vi "Soft_Robot_Model_Conf.vi"() -> ()   [LabVIEW 2015]
uses:
  <vilib>/addons/Control Design/_Stochastic Systems/Stochastic Systems.llb/Stochastic Systems SubVIs/cd_Stochastic State-Space Model.ctl
  <vilib>/addons/Control Design/_Model Construction/Model Typedefs.llb/CD State Space Model (MIMO).ctl
  <vilib>/addons/Control Design/_Model Construction/Model Typedefs.llb/CD General Elements.ctl
  <vilib>/addons/Control Design/_Stochastic Systems/Stochastic Systems.llb/CD CtoD Stochastic Model.ctl
  <vilib>/Platform/TimedLoop/XDataNode/timing_clust.ctl
  <vilib>/Platform/TimedLoop/XDataNode/nitl_modes.ctl
  <vilib>/Platform/TimedLoop/XDataNode/wakeup.ctl
  <vilib>/addons/Control Design/_Stochastic Systems/Stochastic Systems.llb/CD Construct Stochastic Model (Numeric).vi
  <vilib>/FPGAPlugInAG/myRIO-1900/niLvFpga_Open_myRIO-1900.vi
  <vilib>/rvi/interface/common/dynamic/niFpgaDynamicAddResources.vi
  <vilib>/Utility/error.llb/Error Cluster From Error Code.vi
  <vilib>/rvi/errors/niLvFpgaAdjustHostInterfaceError.vi
  <vilib>/FPGAPlugInAG/Dynamic/niLvFpga_Close_Dynamic.vi
  <vilib>/Analysis/7linalg.llb/Create Special Real Matrix.vi
  <vilib>/addons/Control Design/_Stochastic Systems/Stochastic Systems.llb/CD Construct Noise Model (Numeric).vi
  <vilib>/addons/Control Design/_State Feedback Control/State Feedback Control.llb/State Feedback Control SubVis/cd_Linear Quadratic Regulator.vi
  <vilib>/Simulation/Estimation/Implementation/NILVSim Discrete Kalman Filter.llb/SIM Disc KF Pred and Corr with Pred Gain with Checking Direct LV.vi
  <vilib>/Simulation/DiscreteLinear/Implementation/NILVSim Discrete Stochastic State Space.llb/NILVSim Discrete Stochastic State Space Internal Direct LV.vi
  <vilib>/addons/Control Design/_Implementation/CD State Feedback Controller (Multiple Outputs).vi
  <vilib>/Platform/TimedLoop/XDataNode/XDataNode.xnode
  <vilib>/rvi/interface/nirviOpenFPGA/nirviOpenFPGA.xnode
  FPGA Bitfiles/ACC20115_FPGATarget_CurrentControlle_Dt5vFgOzYtY.lvbitx
  Current Controller.vi
  <vilib>/rvi/interface/nirviReadWriteControl/nirviReadWriteControl.xnode
  <vilib>/rvi/interface/nirviCloseFPGA/nirviCloseFPGA.xnode
  <vilib>/Simulation/Implementation/XNodeFramework/SimXNode/SimX.xnode
  <vilib>/addons/Control Design/_State Feedback Control/NI_CD_State Feedback Control.lvlib
  <vilib>/Analysis/NI_AALPro.lvlib
  <vilib>/Platform/TimedLoop/XDataNode/XDNodeRunTimeDep.lvlib
  <vilib>/rvi/interface/Simulation/niFpgaSimulationCallBeginRW.vi
  <vilib>/addons/Control Design/_Stochastic Systems/NI_CD_Stochastic Systems.lvlib
  <vilib>/addons/Control Design/_State-Space Analysis/NI_CD_State-Space Analysis.lvlib
  NiFpgaLv.dll
  <vilib>/addons/Control Design/_Implementation/NI_CD_Implementation.lvlib
  <vilib>/addons/Control Design/_Model Construction/NI_LinSys_Model Typedefs.lvlib
panel:
  in  "SP":dbl(slide) scale=580.0..720.0
  in  "Tab Control":enum32{"Outputs", "SS Outs", "Inputs"}(tab)
  out "Applied Current":i32(graph)
  out "Status?":bool
  out "Is Detectable?":bool
  out "Is Observable?":bool
  out "Is Controllable?":bool
  out "Is Stabilizable?":bool
  out "Fusion":dbl(graph)
  in  "Current (mA)":i32
  out "KF Post":dbl[](graph)
  out "Estimation Error":dbl[][](graph)=[[7.63674958364943e-06]]
  out "Plant Output and KF estimation":dbl[][](graph)=[[0.009100087472457918]]
  out "Filtered State Estimate (Kalman Filter)":dbl[][](graph)
  out "Kalman Predictor Gain L(k)":dbl[][](array[numeric])=[[1.0]] format="%#.6g"
  out "Kalman Filter Gain M(k)":dbl[][](array[numeric]) format="%#.6g"
  in  "Stop":bool
  out "Stochastic State-Space Model":T1={"Sampling Time (s)"=0.0, "G"=[], "B"=[[-1.71e-07], [6.47e-07]], "A"=[], "C"=[], "D"=[], "H"=[]} {"H" format="%#.2g"; "D" format="%#.2g"; "C" format="%#.2g"; "A" format="%#.2g"; "B" format="%#.2g"; "G" format="%#.2g"; "Sampling Time (s)" format="%.2f"}
  out "Deterministic State-Space Model":T2={"properties"={"Model name"="", "Input names"=[], "Output names"=[], "Input Delays"=[], "Output Delays"=[], "Sampling Time"=0.0, "Notes"=""}, "A"=[], "B"=[[-1.706e-07], [6.469e-07]], "C"=[], "D"=[], "StateNames"=[], "Transport Delay"=[]} {"Transport Delay" format="%.2f"; "D" format="%#.2g"; "C" format="%#.2g"; "B" format="%#.2g"; "A" format="%#.2g"; "properties"."Sampling Time" format="%#.6p"; "properties"."Output Delays" format="%.4f"; "properties"."Input Delays" format="%.4f"}
  out "error out":errorcluster
  out "LQR Error":errorcluster
  in  "LQR Matrix (Q)":dbl[](array[slide])=[10000000000.00004, 667179.0862882147, 4641588833.612801] scale=0.001..1e+16
  in  "LQR Output  matrix (R)":dbl[](array[slide])=[0.09999999999999994] scale=0.001..10.0
  in  "A":dbl[][](array[numeric])=[[1.01, -0.1716], [0.001556, 0.9782]] format="%#.5g"
  in  "B":dbl[][](array[numeric])=[[-1.706e-07], [6.469e-07]] format="%#.5g"
  in  "C":dbl[][](array[numeric])=[[1.089, -0.03769]] format="%#.5g"
  out "LQR Eigenvalues":cdb[](array[numeric]) format="%.5f"
  in  "G":dbl[][](array[numeric])=[[0.9253], [0.9604]] format="%#.2g"
  in  "xhat(0|-1)":dbl[](array[numeric])=[1.0, 0.0]
  in  "P(0|-1)":dbl[][](array[numeric])=[[1.0, 0.0], [0.0, 1.0]]
  in  "KF Q":dbl[](array[slide])=[10000000000.00004, 0.5250344735515627] scale=0.001..5000.0
  in  "KF R":dbl[](array[slide])=[24.170001062768083, 1.5278416161534805] scale=0.001..5000.0
  in  "KF Q/R Size":i32=2
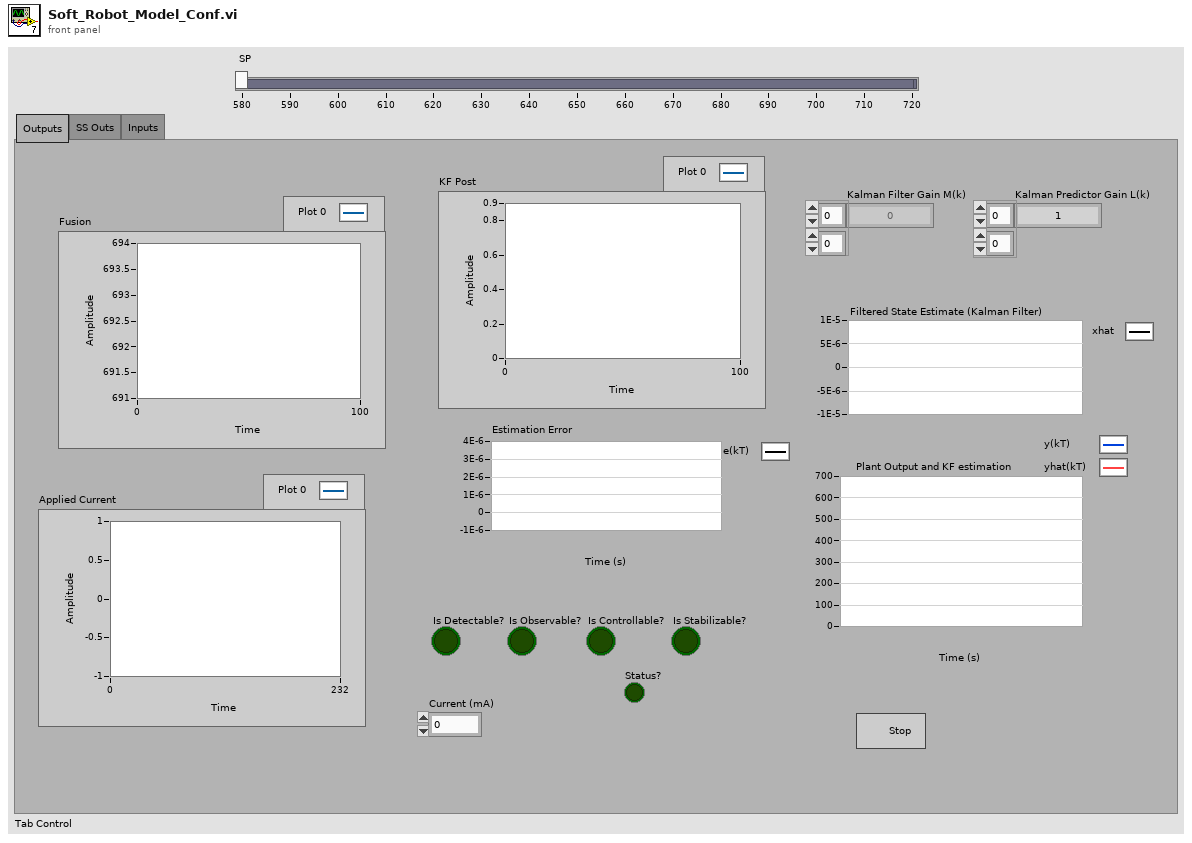
[diagram p1: front panel]
types:
  T1 = typedef "NI_CD_Stochastic Systems.lvlib/cd_Stochastic State-Space Model.ctl" = cluster{"Sampling Time (s)":dbl, "G":dbl[][], "B":dbl[][], "A":dbl[][], "C":dbl[][], "D":dbl[][], "H":dbl[][]}
  T2 = typedef "NI_LinSys_Model Typedefs.lvlib/CD State Space Model (MIMO).ctl" = cluster{"properties":T3, "A":dbl[][], "B":dbl[][], "C":dbl[][], "D":dbl[][], "StateNames":string[], "Transport Delay":dbl[][]}
  T3 = typedef "NI_LinSys_Model Typedefs.lvlib/CD General Elements.ctl" = cluster{"Model name":string, "Input names":string[], "Output names":string[], "Input Delays":dbl[], "Output Delays":dbl[], "Sampling Time":dbl, "Notes":string}
  T4 = typedef "NI_CD_Stochastic Systems.lvlib/CD CtoD Stochastic Model.ctl" = enum16{"Truncation of Taylor Series", "Numerical Integration"}
  T5 = typedef "XDNodeRunTimeDep.lvlib/timing_clust.ctl" = cluster{"Expected End [f-1]":u64, "Actual End [f-1]":u64, "Finished Late? [f-1]":bool, "Expected End [i-1]":u64, "Actual End [i-1]":u64, "Finished Late? [i-1]":bool, "Expected Start [i]":u64, "Actual Start [i]":u64, "Expected Start [f]":u64, "Actual Start [f]":u64, "Source Name":string, "Structure Name":string, "Period":i64, "Deadline":i64, "Offset":i64, "Start":i64, "Priority":i32, "Timeout":i32, "Mode":T6, "Wakeup Reason":T7, "Error":errorcluster, "Source Type":string, "Secondary Source Type":string, "Global End Time":u64, "Global Start Time":u64, "Frame Duration":u64, "Iteration Duration":u64, "Assigned CPU":i32, "I/O Scan Engine Mode":u32}
  T6 = typedef "XDNodeRunTimeDep.lvlib/nitl_modes.ctl" = enum32{"No Change", "Process missed periods, maintain original phase", "Discard missed periods, maintain original phase", "Process missed periods, ignore original phase", "Discard missed periods, ignore original phase"}
  T7 = typedef "XDNodeRunTimeDep.lvlib/wakeup.ctl" = enum32{"Normal", "Aborted", "Asynchronous wakeup", "Timing source error", "Timed loop error", "Timeout"}
  T8 = typedef "NI_Matrix.lvlib/RealMatrix.ctl" = dbl[][]
  T9 = typedef "NI_CD_Stochastic Systems.lvlib/cd_Second-Order Statistics Noise Model.ctl" = cluster{"Q":dbl[][], "E{w}":dbl[], "E{v}":dbl[], "R":dbl[][], "N":dbl[][]}
  T10 = enum16{"state weighting", "output weighting, Dim Q = Ny", "output weighting, Dim Q = Nx"}
  T11 = enum32{"Identity", "Diagonal", "Toepliz", "Vandermonde", "Companion"}
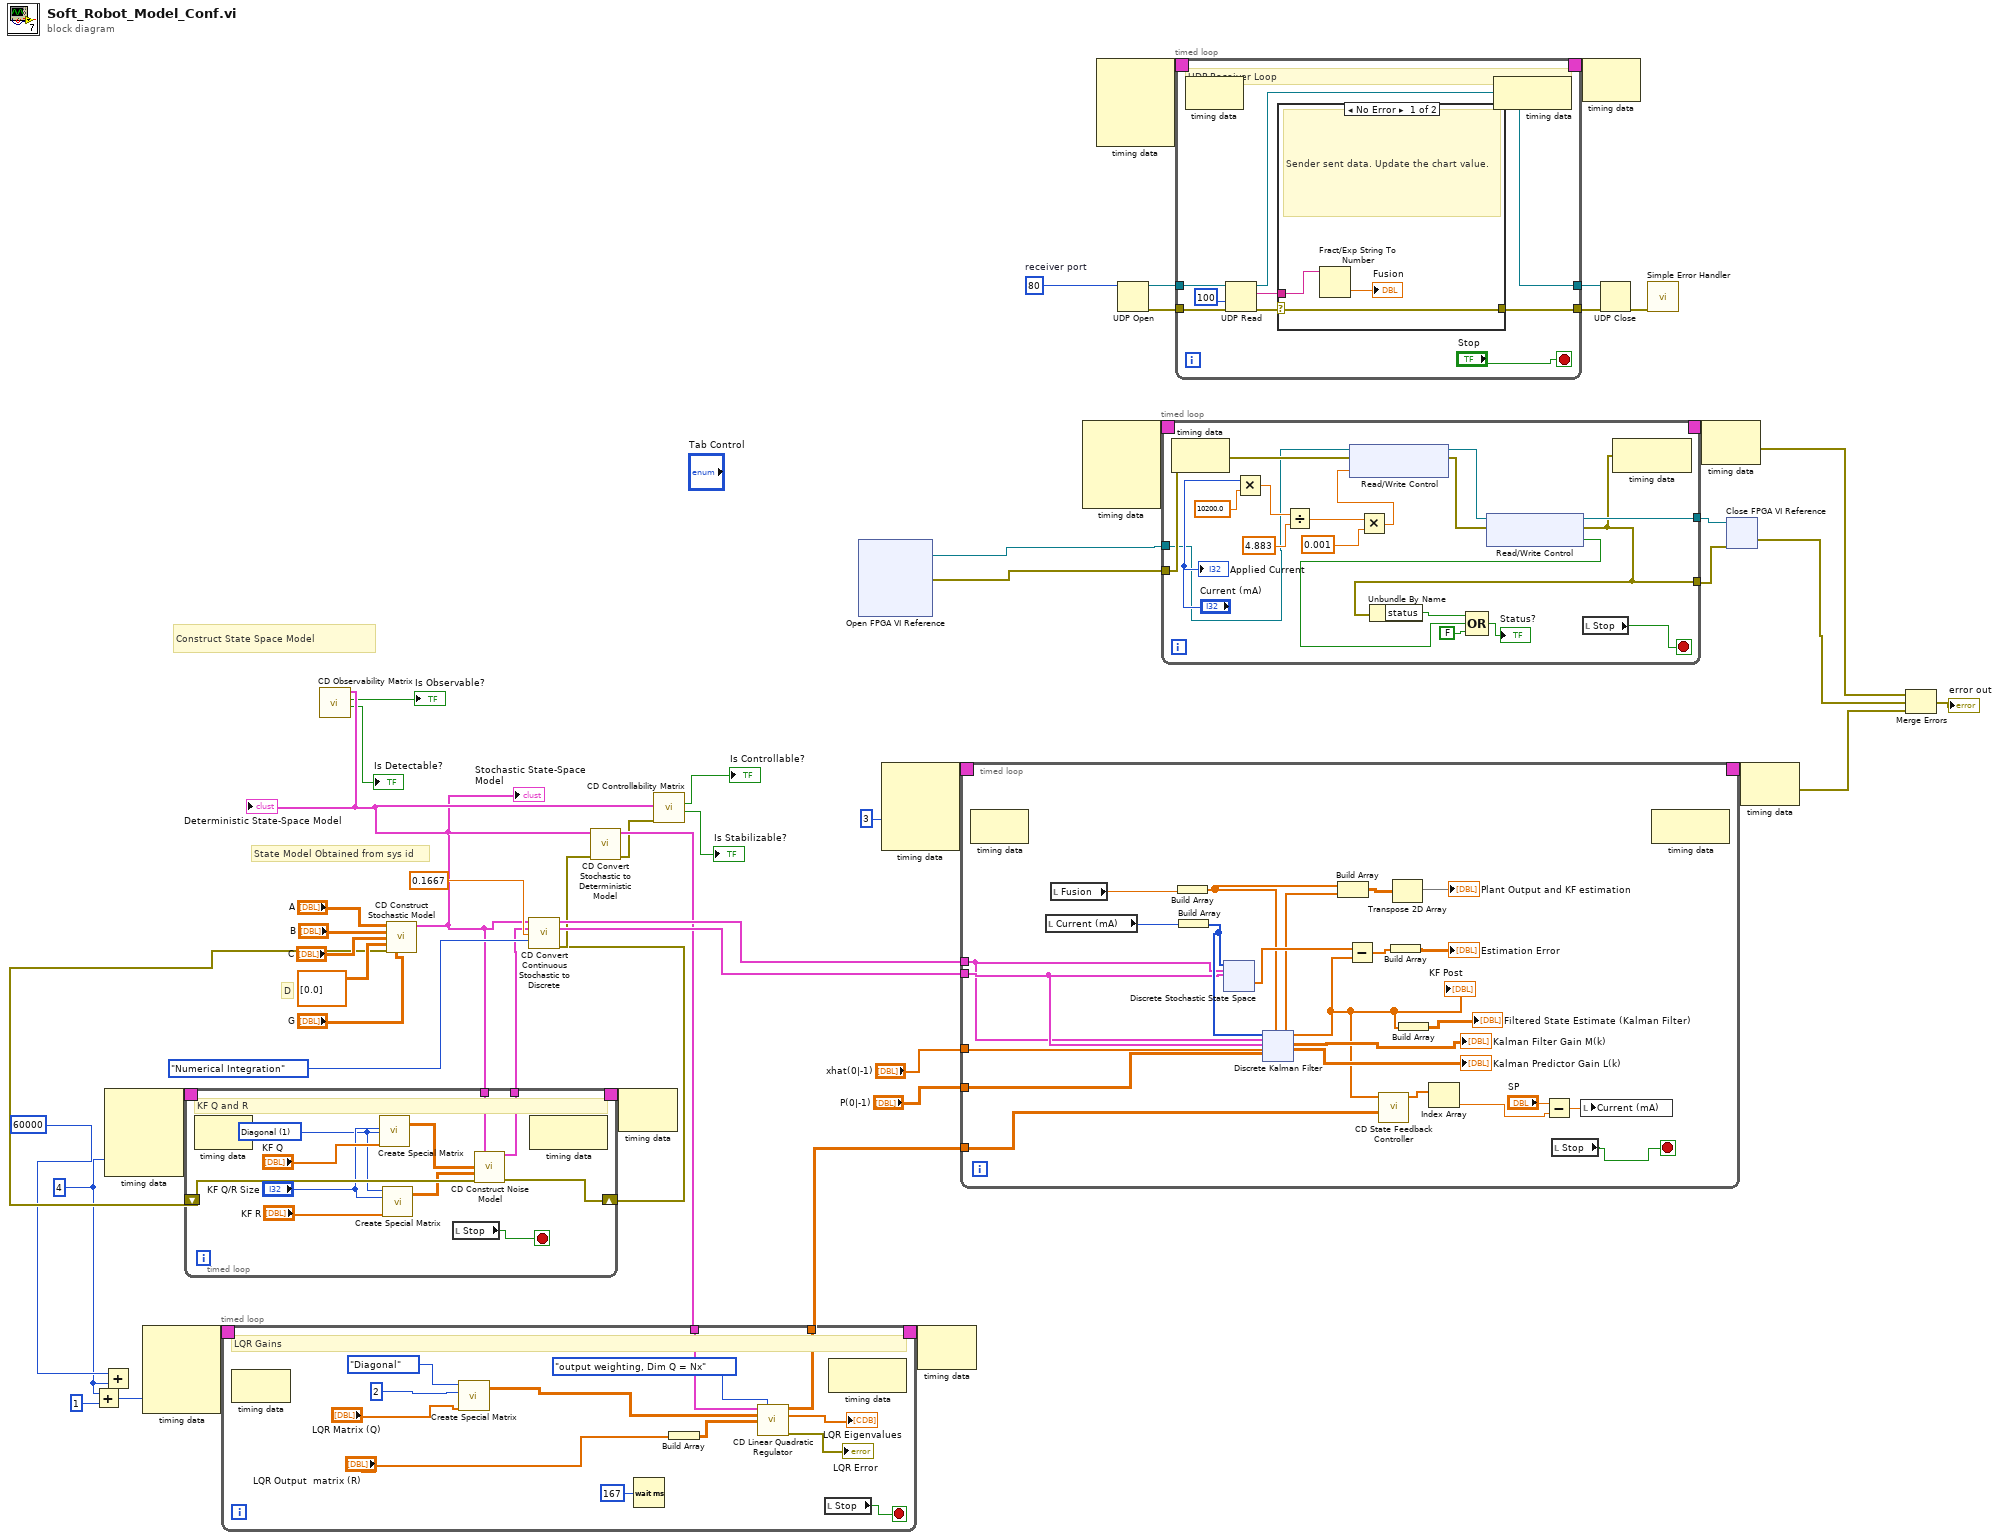
[diagram p0: block diagram]
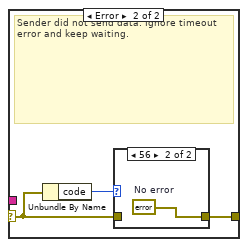
[diagram p2: hidden frame]
diagram:
  w2 = 4 ("Processor")
  w36 = u16 80  # receiver port
  # "D"
  # "State Model Obtained from sys id"
  # "Construct State Space Model"
  n1 = Add(x=w2, y=1) -> (x+y=w3:i32)
  n2 = Add(x=60000 ("Priority"), y=w2) -> ()  [unwired: 1 out]
  n3 = node-c288(w2) -> (w7:T5)  [unwired: 3 in]
  n4 = node-c288(w3) -> (w5:T5)  [unwired: 3 in]
  n5 = call-poly <vilib>:"CD Construct Stochastic Model.vi"("A"="A", "B"="B", "C"="C", "D"=dbl[][] [[0.0]], "G"="G") -> ("Stochastic State-Space Model"=w22:T1, "error out"=w15:errorcluster)  [unwired: 3 in, 6 out]
  "Stochastic State-Space Model" <- w22
  n6 = timed-loop {
    tunnel: [w63] -> w23
    tunnel: w22 -> [w62]
    shift-right: [w60] -> w14
    shift-left: w15 -> [w61]
    timing: w7 -> [_]
    timing-out: [_] -> w6
    stop <- w53 stop-if-true
    w54 = 1 items=["Identity", "Diagonal", "Toeplitz", "Vandermonde", "Companion", "Hankel", "Hadamard", "Wilkinson", "Hilbert", "Inverse Hilbert", "Rosser", "Pascal"] ("matrix type")
    # "KF Q and R"
    n7 = node-c288() -> ()  [unwired: 1 in, 1 out]
    n8 = call-poly <vilib>:"Create Special Matrix.vi"("matrix type"=w54, "matrix size"="KF Q/R Size", "Input Vector1"="KF Q") -> ("Special Matrix"=w59:T8)  [unwired: 2 in, 1 out]
    n9 = call-poly <vilib>:"Create Special Matrix.vi"("matrix type"=w54, "matrix size"="KF Q/R Size", "Input Vector1"="KF R") -> ("Special Matrix"=w58:T8)  [unwired: 2 in, 1 out]
    n10 = local read "Stop"() -> (w53:bool)
    n11 = call-poly <vilib>:"CD Construct Noise Model.vi"("Stochastic State-Space Model"=w62, "Q"=w59, "R"=w58, "error in (no error)"=w61) -> ("Second-Order Statistics Noise Model out"=w63:T9, "error out"=w60:errorcluster)  [unwired: 3 in, 7 out]
    n12 = node-c288() -> ()  [unwired: 1 in, 1 out]
  }
  n13 = call <vilib>:"CD Convert Continuous Stochastic to Discrete.vi"("Continuous Stochastic\nState-Space Model"=w22, "Continuous Second-Order\nStatistics Noise Model"=w23, "Sampling Time (s)"=0.1667, "Method"=CD_CtoD_Stochastic_Model."Numerical Integration", "error in (no error)"=w14) -> ("Discrete Stochastic\nState-Space Model"=w43:T1, "Discrete Second-Order\nStatistics Noise Model"=w44:T9, "error out"=w17:errorcluster)  [unwired: 8 out]
  n14 = call <vilib>:"CD Convert Stochastic to Deterministic Model.vi"("Stochastic State-Space Model"=w22, "error in (no error)"=w17) -> ("Deterministic State-Space Model"=w42:T2, "error out"=w16:errorcluster)  [unwired: 12 in]
  "Deterministic State-Space Model" <- w42
  n15 = timed-loop {
    tunnel: [w74] -> w48
    tunnel: w42 -> [w72]
    timing: w5 -> [_]
    timing-out: [_] -> w4
    stop <- w67 stop-if-true
    # "LQR Gains"
    n16 = node-c288() -> ()  [unwired: 1 in, 1 out]
    n17 = call-poly <vilib>:"Create Special Matrix.vi"("matrix type"=T11."Diagonal", "matrix size"=2, "Input Vector1"="LQR Matrix (Q)") -> ("Special Matrix"=w75:T8)  [unwired: 2 in, 1 out]
    n18 = Wait (ms)(milliseconds to wait=u32 167) -> ()  [unwired: 1 out]
    n19 = Build Array("LQR Output  matrix (R)") -> (w71:dbl[][])
    n20 = call-poly <vilib>:"CD Linear Quadratic Regulator.vi"("State-Space Model"=w72, "Weighting Type"=T10."output weighting, Dim Q = Nx", "Q"=w75, "R"=w71) -> ("Optimal Gain (K)"=w74:dbl[][], "Eigenvalues"=→"LQR Eigenvalues":cdb[], "error out"=→"LQR Error":errorcluster)  [unwired: 8 in, 1 out]
    n21 = local read "Stop"() -> (w67:bool)
    n22 = node-c288() -> ()  [unwired: 1 in, 1 out]
  }
  n23 = call <vilib>:"CD Observability Matrix.vi"("State-Space Model"=w42) -> ("Is Detectable?"=→"Is Detectable?":bool, "Is Observable?"=→"Is Observable?":bool)  [unwired: 7 in, 2 out]
  n24 = node-c288(w6) -> ()  [unwired: 1 out]
  n25 = call <vilib>:"CD Controllability Matrix.vi"("error in (no error)"=w16, "State-Space Model"=w42) -> ("Is Stabilizable?"=→"Is Stabilizable?":bool, "Is Controllable?"=→"Is Controllable?":bool)  [unwired: 6 in, 2 out]
  n26 = xnode "Open FPGA VI Reference"() -> ("FPGA VI Reference Out"=w35:refnum<k20>, "error out"=w34:errorcluster)  [unwired: 2 in]
  n27 = node-c288(3 ("Processor")) -> (w33:T5)  [unwired: 3 in]
  n28 = node-c288(w4) -> ()  [unwired: 1 out]
  n29 = timed-loop {
    timing: w33 -> [_]
    timing-out: [_] -> w32
    tunnel: w48 -> [w89]
    tunnel: w44 -> [w88]
    tunnel: w43 -> [w87]
    tunnel: "xhat(0|-1)" -> [w86]
    tunnel: "P(0|-1)" -> [w85]
    stop <- w81 stop-if-true
    n30 = node-c288() -> ()  [unwired: 1 in, 1 out]
    n31 = local read "Current (mA)"() -> (w82:i32)
    n32 = local read "Fusion"() -> (w83:dbl)
    n33 = Build Array ("Build Array 3")(w83) -> (w93:dbl[])
    n34 = Build Array ("Build Array 5")(w82) -> (w103:i32[])
    n35 = xnode ("Discrete Stochastic State Space")("Input u(k)"=w103, "Stochastic State-Space Model"=w87, "Second-Order Statistics Noise Model"=w88) -> ("State x(k)"=w102:dbl[])  [unwired: 3 in, 3 out]
    n36 = xnode ("Discrete Kalman Filter")("input u(k)"=w103, "Stochastic State-Space Model"=w87, "Second-Order Statistics Noise Model"=w88, "Initial State Estimate xhat(0|-1)"=w86, "Initial Estimation Error Covariance P(0|-1)"=w85, "Output y(k)"=w93) -> ("Estimated Output yhat(k)"=w99:dbl[], "Corrected State Estimate xhat(k|k)"=w94:dbl[], "Kalman Filter Gain M(k)"=→"Kalman Filter Gain M(k)":dbl[][], "Kalman Predictor Gain L(k)"=→"Kalman Predictor Gain L(k)":dbl[][])  [unwired: 2 in, 4 out]
    "KF Post" <- w94
    n37 = Build Array(w93, w99) -> (w98:dbl[][])
    n38 = Subtract(x=w102, y=w94) -> (x-y=w101:dbl[])
    n39 = call-poly <vilib>:"CD State Feedback Controller.vi"("Controller Gain"=w89, "States"=w94) -> ("Controller Action"=w104:dbl[])  [unwired: 8 in, 1 out]
    n40 = Build Array ("Build Array 6")(w101) -> (→"Estimation Error":dbl[][])
    n41 = Transpose 2D Array(2D array=w98) -> (transposed array=→"Plant Output and KF estimation":dbl[][])
    n42 = Build Array ("Build Array 2")(w94) -> (→"Filtered State Estimate (Kalman Filter)":dbl[][])
    n43 = Index Array(array=w104) -> (element=w90:dbl)  [unwired: 1 in]
    n44 = Subtract ("Subtract 2")(x="SP", y=w90) -> (x-y=w84:dbl)
    n45 = local read "Stop"() -> (w81:bool)
    n46 = local write "Current (mA)"(w84) -> ()
    n47 = node-c288() -> ()  [unwired: 1 in, 1 out]
  }
  n48 = node-c288() -> (w50:T5)  [unwired: 4 in]
  n49 = node-c288() -> (w9:T5)  [unwired: 4 in]
  n50 = UDP Open(11:w36) -> (port=w37:refnum<k16>, 0:w38:errorcluster)  [unwired: 4 in, 1 out]
  n51 = timed-loop {
    tunnel: w34 -> [w136]
    tunnel: [w135] -> w47
    tunnel: [w144] -> w52
    timing: w50 -> [_]
    timing-out: [_] -> w49
    tunnel: w35 -> [w134]
    stop <- w133 stop-if-true
    n52 = node-c288() -> ()  [unwired: 1 in, 1 out]
    n53 = Multiply(x="Current (mA)", y=10200.0) -> (x*y=w139:dbl)
    n54 = Divide(x=w139, y=4.883) -> (x/y=w142:dbl)
    n55 = Multiply(x=w142, y=0.001) -> (x*y=w138:dbl)
    n56 = xnode "Read/Write Control"("FPGA VI Reference In"=w134, "error in"=w136, "DAC Inlet Valve"=w138) -> ("FPGA VI Reference Out"=w150:refnum<k20>, "error out"=w149:errorcluster)
    n57 = xnode "Read/Write Control"("FPGA VI Reference In"=w150, "error in"=w149) -> ("FPGA VI Reference Out"=w144:refnum<k20>, "error out"=w135:errorcluster, "Inlet Overflow?"=w145:bool)
    n58 = Unbundle By Name(w135) -> ("status"=w147:bool)
    n59 = Compound Arithmetic op=OR(w147, w145, FALSE ("value")) -> (→"Status?":bool)
    n60 = local read "Stop"() -> (w133:bool)
    n61 = node-c288(w135) -> ()  [unwired: 1 out]
    "Applied Current" <- "Current (mA)"
  }
  n62 = timed-loop {
    tunnel: w37 -> [w162]
    tunnel: [w156] -> w41
    tunnel: w38 -> [w161]
    tunnel: [w157] -> w39
    timing: w9 -> [_]
    timing-out: [_] -> w8
    stop <- "Stop" stop-if-true
    # "UDP Receiver Loop"
    n63 = node-c288() -> ()  [unwired: 1 in, 1 out]
    n64 = UDP Read(connection ID=w162, timeout ms (25000)=100, 8:w161) -> (data out=w159:string, error out=w158:errorcluster, 3:w156:refnum<k16>)  [unwired: 3 out]
    n65 = case shown="No Error" w158 {
      selector: w158 -> [w165 w169]
      tunnel: w159 -> [w167 _]
      tunnel: [w165 w168] -> w157
      frame No Error {
        # "Sender sent data. Update the chart value."
        n66 = Fract/Exp String To Number(string=w167) -> (number=→"Fusion":dbl)  [unwired: 3 in, 1 out]
      }
      frame Error {
        # "Sender did not send data. Ignore timeout error and keep waiting."
        n67 = Unbundle By Name(w169) -> ("code"=w170:i32)
        n68 = case shown="56" w170 {
          tunnel: w169 -> [w171 _]
          tunnel: [w171 w172] -> w168
          frame Default {
          }
          frame 56 {
            w172 = errorcluster {"status"=FALSE, "code"=0, "source"=""}  # No error
          }
        }
      }
    }
    n69 = node-c288() -> ()  [unwired: 1 in, 1 out]
  }
  n70 = node-c288(w8) -> ()  [unwired: 1 out]
  n71 = UDP Close(connection ID=w41, 8:w39) -> (error out=w40:errorcluster)  [unwired: 1 out]
  n72 = call <vilib>:"Simple Error Handler.vi"("error in (no error)"=w40) -> ()  [unwired: 1 in, 8 out]
  n73 = node-c288(w49) -> (w45:errorcluster)
  n74 = xnode "Close FPGA VI Reference"("FPGA VI Reference In"=w52, "error in"=w47) -> ("error out"=w46:errorcluster)
  n75 = node-c288(w32) -> (w12:errorcluster)
  n76 = Merge Errors(w45, w46, w12) -> (→"error out":errorcluster)
